vi "Ls372_Merge_Cluster.vi"(1 "LS372-Control":T2 {"MC Thermometer" items=["Speer 9905", "ROX U02453"]}, 2 "LS372-Status":T1) -> (0 "LS372-Cluster":T3 {"MC Thermometer" items=["Speer 9905", "ROX U02453"]})   [LabVIEW 2019]
uses:
  LS372/LS372-Cluster.ctl
  LS372/Ls372-Control.ctl
  LS372/LS372-Status.ctl
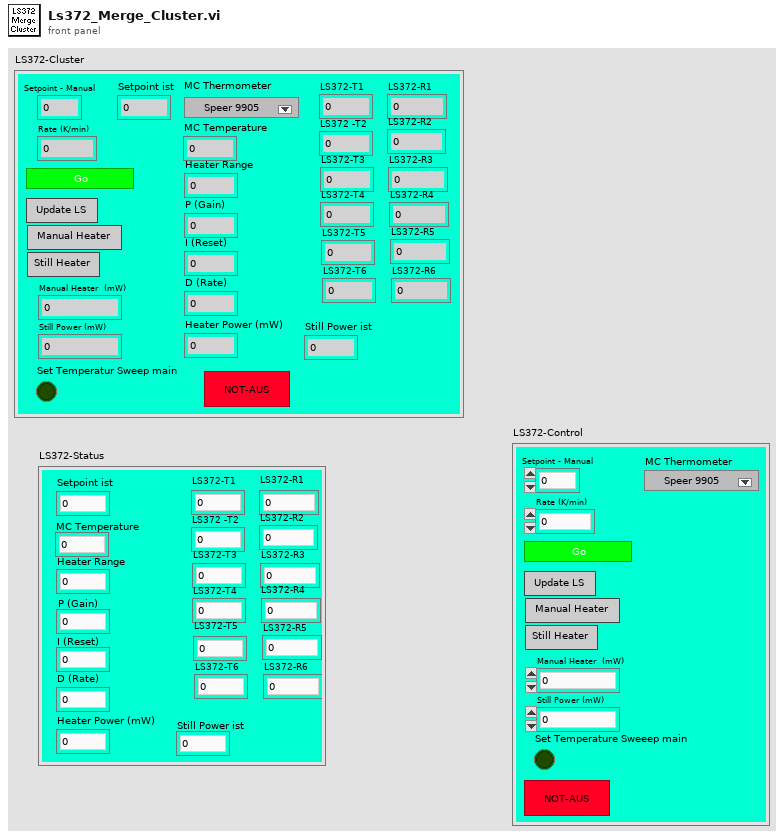
[diagram p1: front panel]
types:
  T1 = typedef "LS372-Status.ctl" = cluster{"Heater Range":dbl, "P (Gain)":dbl, "I (Reset)":dbl, "D (Rate)":dbl, "Heater Power (mW)":dbl, "MC Temperature":dbl, "LS372-T1":dbl, "LS372 -T2":dbl, "LS372-R1 ":dbl, "LS372-R2":dbl, "LS372-T3":dbl, "LS372-T4":dbl, "LS372-R3 ":dbl, "LS372-R4 \n\n\n\n":dbl, "LS372-T5":dbl, "LS372-T6":dbl, "LS372-R5":dbl, "LS372-R6 ":dbl, "Still Power ist":dbl, "Setpoint ist":dbl}
  T2 = typedef "Ls372-Control.ctl" = cluster{"Activate Tsweep":bool, "Setpoint - Manual":dbl, "Rate (K/min)":dbl, "Update Lakeshores":bool, "Still Heater":bool, "Still Power (mW)":dbl, "Manual Heater":bool, "Manual Heater  (mW) ":dbl, "MC Thermometer":u16, "Set Temperature Sweeep main":bool, "Disable Heater":bool}
  T3 = typedef "LS372-Cluster.ctl" = cluster{"Activate Tsweep":bool, "Setpoint - Manual":dbl, "Rate (K/min)":dbl, "Update Lakeshores":bool, "Still Heater":bool, "Still Power (mW)":dbl, "Manual Heater":bool, "Manual Heater  (mW) ":dbl, "Heater Range":dbl, "P (Gain)":dbl, "I (Reset)":dbl, "D (Rate)":dbl, "Heater Power (mW)":dbl, "MC Thermometer":u16, "MC Temperature":dbl, "LS372-T1":dbl, "LS372 -T2":dbl, "LS372-R1 ":dbl, "LS372-R2":dbl, "LS372-T3":dbl, "LS372-T4":dbl, "LS372-R3 ":dbl, "LS372-R4 \n\n\n\n":dbl, "LS372-T5":dbl, "LS372-T6":dbl, "LS372-R5":dbl, "LS372-R6 ":dbl, "Still Power ist":dbl, "Set Temperatur Sweep main":bool, "Setpoint ist":dbl, "Disable Heater":bool}
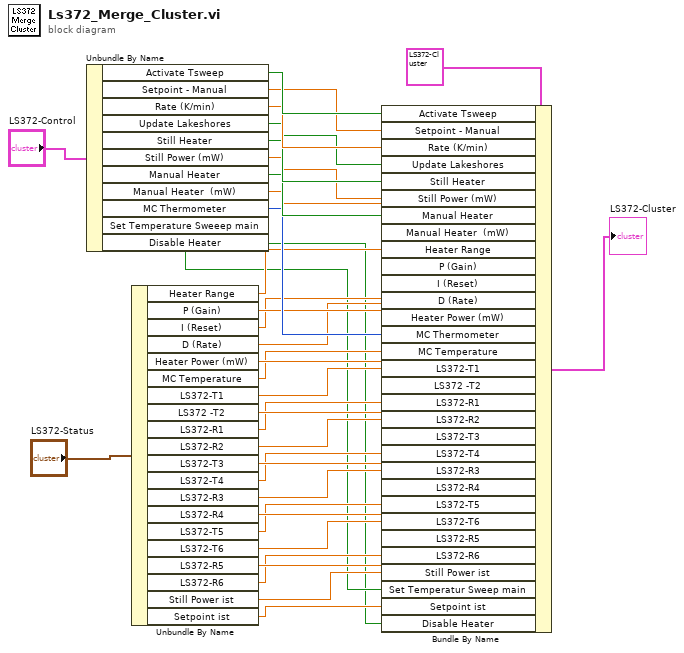
[diagram p0: block diagram]
diagram:
  n1 = Unbundle By Name("LS372-Control") -> ("Activate Tsweep"=w31:bool, "Setpoint - Manual"=w30:dbl, "Rate (K/min)"=w29:dbl, "Update Lakeshores"=w28:bool, "Still Heater"=w27:bool, "Still Power (mW)"=w26:dbl, "Manual Heater"=w25:bool, "Manual Heater  (mW)"=w24:dbl, "MC Thermometer"=w23:u16, "Set Temperature Sweeep main"=w3:bool, "Disable Heater"=w1:bool)
  n2 = Unbundle By Name("LS372-Status") -> ("Heater Range"=w22:dbl, "P (Gain)"=w21:dbl, "I (Reset)"=w20:dbl, "D (Rate)"=w19:dbl, "Heater Power (mW)"=w18:dbl, "MC Temperature"=w17:dbl, "LS372-T1"=w16:dbl, "LS372 -T2"=w15:dbl, "LS372-R1"=w14:dbl, "LS372-R2"=w13:dbl, "LS372-T3"=w12:dbl, "LS372-T4"=w11:dbl, "LS372-R3"=w10:dbl, "LS372-R4"=w9:dbl, "LS372-T5"=w8:dbl, "LS372-T6"=w7:dbl, "LS372-R5"=w6:dbl, "LS372-R6"=w5:dbl, "Still Power ist"=w4:dbl, "Setpoint ist"=w2:dbl)
  n3 = Bundle By Name(cluster=T3 {"Activate Tsweep"=FALSE, "Setpoint - Manual"=0.0, "Rate (K/min)"=0.0, "Update Lakeshores"=FALSE, "Still Heater"=FALSE, "Still Power (mW)"=0.0, "Manual Heater"=FALSE, "Manual Heater  (mW) "=0.0, "Heater Range"=0.0, "P (Gain)"=0.0, "I (Reset)"=0.0, "D (Rate)"=0.0, "Heater Power (mW)"=0.0, "MC Thermometer"=0, "MC Temperature"=0.0, "LS372-T1"=0.0, "LS372 -T2"=0.0, "LS372-R1 "=0.0, "LS372-R2"=0.0, "LS372-T3"=0.0, "LS372-T4"=0.0, "LS372-R3 "=0.0, "LS372-R4 \n\n\n\n"=0.0, "LS372-T5"=0.0, "LS372-T6"=0.0, "LS372-R5"=0.0, "LS372-R6 "=0.0, "Still Power ist"=0.0, "Set Temperatur Sweep main"=FALSE, "Setpoint ist"=0.0, "Disable Heater"=FALSE} ("LS372-Cluster 2"), "Activate Tsweep"=w31, "Setpoint - Manual"=w30, "Rate (K/min)"=w29, "Update Lakeshores"=w28, "Still Heater"=w27, "Still Power (mW)"=w26, "Manual Heater"=w25, "Manual Heater  (mW)"=w24, "Heater Range"=w22, "P (Gain)"=w21, "I (Reset)"=w20, "D (Rate)"=w19, "Heater Power (mW)"=w18, "MC Thermometer"=w23, "MC Temperature"=w17, "LS372-T1"=w16, "LS372 -T2"=w15, "LS372-R1"=w14, "LS372-R2"=w13, "LS372-T3"=w12, "LS372-T4"=w11, "LS372-R3"=w10, "LS372-R4"=w9, "LS372-T5"=w8, "LS372-T6"=w7, "LS372-R5"=w6, "LS372-R6"=w5, "Still Power ist"=w4, "Set Temperatur Sweep main"=w3, "Setpoint ist"=w2, "Disable Heater"=w1) -> (→"LS372-Cluster":T3)
